vi "TCPReadWithSize.vi"(8 "error in (no error)":errorcluster, 10 "Timeout ms":i32, 11 "Connection In":refnum<k5>) -> (0 "error out":errorcluster, 2 "Command String":string, 3 "Connection out":refnum<k5>)   [LabVIEW 2015]
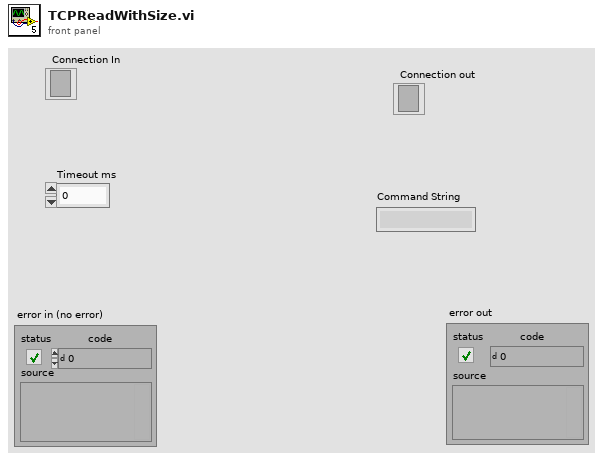
[diagram p1: front panel]
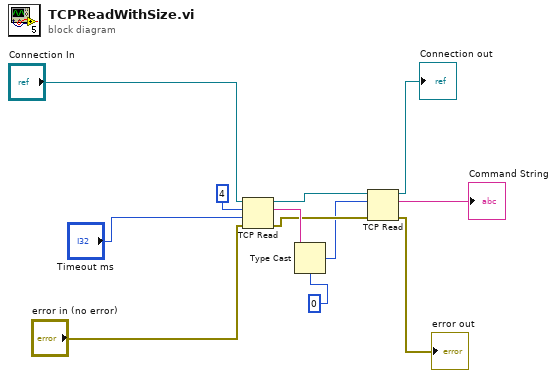
[diagram p0: block diagram]
diagram:
  n1 = TCP Read(connection ID="Connection In", bytes to read=4, error in (no error)="error in (no error)", 9:"Timeout ms") -> (connection ID out=w5:refnum<k5>, data out=w9:string, error out=w8:errorcluster)  [unwired: 1 in]
  n2 = Type Cast(type=u32 0, x=w9) -> (*(type *) &x=w6:u32)
  n3 = TCP Read(connection ID=w5, bytes to read=w6, error in (no error)=w8) -> (connection ID out=→"Connection out":refnum<k5>, data out=→"Command String":string, error out=→"error out":errorcluster)  [unwired: 2 in]
